vi "registro-usuario.vi"() -> ()   [LabVIEW 2024]
uses:
  <vilib>/Utility/file.llb/Write Delimited Spreadsheet (string).vi
panel:
  in  "stop":bool
  in  "registrButt":bool
  in  "Registrar Usuario":T1
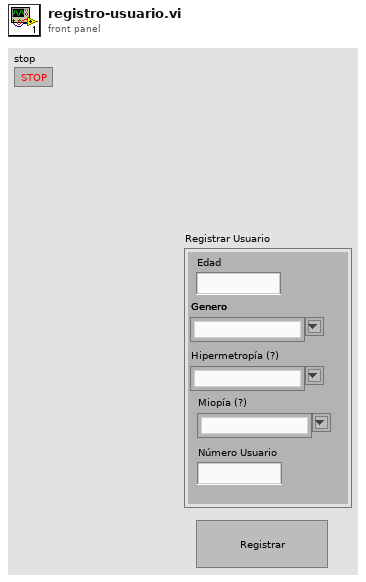
[diagram p1: front panel]
types:
  T1 = cluster{"Miopía (?) ":string, "Hipermetropía (?)":string, "Número Usuario":string, "Edad":string, "Genero":string}
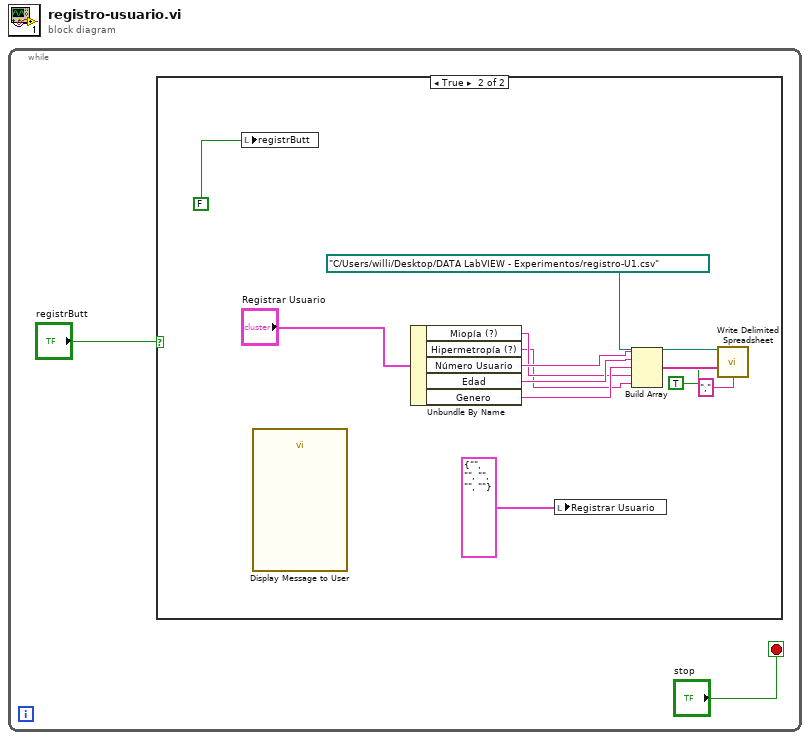
[diagram p0: block diagram]
diagram:
  n1 = while {
    stop <- "stop" stop-if-true
    n2 = case shown="True" "registrButt" {
      frame False {
      }
      frame True {
        n3 = local write "registrButt"(FALSE) -> ()
        n4 = call "Display Message to User"() -> ()  [unwired: 10 in, 2 out]
        n5 = Unbundle By Name("Registrar Usuario") -> ("Miopía (?)"=w5:string, "Hipermetropía (?)"=w4:string, "Número Usuario"=w8:string, "Edad"=w7:string, "Genero"=w6:string)
        n6 = local write "Registrar Usuario"(T1 {"Miopía (?) "="", "Hipermetropía (?)"="", "Número Usuario"="", "Edad"="", "Genero"=""} ("Registrar Usuario")) -> ()
        n7 = Build Array(w8, w7, w6, w5, w4) -> (w13:string[])
        n8 = call-poly <vilib>:"Write Delimited Spreadsheet.vi"("file path (dialog if empty)"=path "C:/Users/willi/Desktop/DATA LabVIEW - Experimentos/registro-U1.csv", "1D data"=w13, "append to file? (new file:F)"=TRUE, "delimiter (\\t)"="," ("delimiter (\\t)")) -> ()  [unwired: 10 in, 2 out]
      }
    }
  }
